vi "Plugin Wrapper Subpanel.vi"() -> ()   [LabVIEW 2021, in "CIF Manager UI.lvlib"]
uses:
  CIF Manager UI.lvlib
  <vilib>/CIF Foundation/CIF Core/CIFUI/Typedef/Run Listen Button.ctl
  CIFManagerUI Class/Typedef/Class Data for Manager SubPanel.ctl
  <vilib>/CIF Foundation/CIF Core/CIFUI/Typedef/Class Data for SubPanel.ctl
  <vilib>/CIF Foundation/CIF Core/CIFUI/Typedef/Core UI References.ctl
  <vilib>/CIF Foundation/CIF Core/CIFUI/Typedef/SubPanel Events.ctl
  <vilib>/CIF Foundation/CIF Core/CIFUI/Typedef/New Connection Plugin Event Data.ctl
  CIFManagerUI Class/Typedef/Core Manager UI References.ctl
  CIFManagerUI Class/Typedef/Channel Connection.ctl
  CIFManagerUI Class/Typedef/New Plugin.ctl
  CIFManagerUI Class/Typedef/CIF_Manager_UI_Tab.ctl
  CIFPluginManager/typedef/New Connection Event Data.ctl
  <vilib>/gRPC/LabVIEW gRPC Library/Shared/grpcId.ctl
  CIFManagerUI Class/CIF_Manager_UI.lvclass/CIF_Manager_UI.ctl
  <vilib>/CIF Foundation/CIF Core/CIFUI/CIF_UI.lvclass/CIF_UI.ctl
  <vilib>/CIF Foundation/CIF Core/CIFUI/Accessors/Read Plugin Connection Map.vi
  <vilib>/CIF Foundation/CIF Core/CIFUI/Accessors/Read Plugin Subpanel Map.vi
  <vilib>/CIF Foundation/CIF Core/CIFUI/SubVIs/Check Run Command Timer.vi
  <vilib>/CIF Foundation/CIF Core/CIFUI/Utilities/Get Human Readable Error.vi
  <vilib>/CIF Foundation/CIF Utilities/Errors/Append Error Location.vi
  <vilib>/CIF Foundation/CIF Core/CIFUI/Accessors/Read Instrument Studio.vi
  CIFManagerUI Class/CIF_Manager_UI.lvclass
  C:/Program Files/National Instruments/LabVIEW 2021/vi.lib/CIF Foundation/CIF Core/CIFUI/CIF_UI.lvclass
  <vilib>/CIF Foundation/CIF Core/CIFUI/UI Helpers/UI Element Update/Empty Tree by Reference.vi
  CIFManagerUI Class/Manager Functions/SubVIs/Initialize Manager Tab by Reference.vi
  <vilib>/CIF Foundation/CIF Core/CIFUI/UI Helpers/UI Element Update/Empty Table by Reference.vi
  CIFManagerUI Class/Wrapper/Close Plugin SubPanel.vi
  <vilib>/CIF Foundation/CIF Utilities/Errors/Human Readable Error Message.vi
  <vilib>/CIF Foundation/CIF Core/CIFUI/CIF_UI.lvclass
  <vilib>/CIF Foundation/CIF Core/CIFCore/Grpc/CIFCoreWrapper/CIFCoreWrapper.lvlib
  <vilib>/gRPC/LabVIEW gRPC Library/grpc-lvsupport-release.lvlib
panel:
  in  "Class Data for Manager SubPanel":T1
  in  "Plugin Selection":u16(ring) items=["tag"]
  in  "Run Listen":T7
  in  "Unload":bool
  in  "Refresh Button":bool
  in  "Plugin Status":string[][](table)
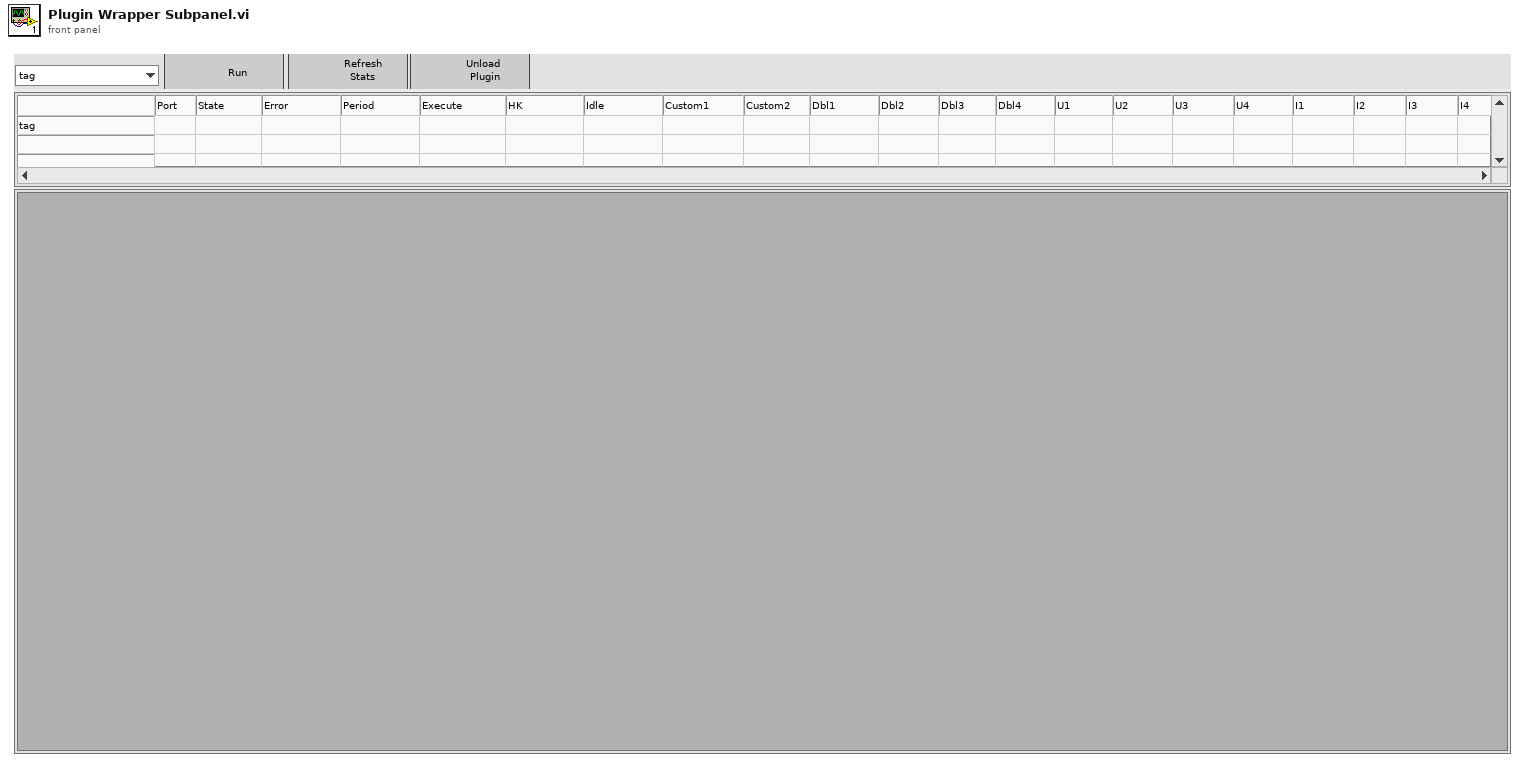
[diagram p1: front panel]
types:
  T1 = typedef "CIF_Manager_UI.lvclass/Class Data for Manager SubPanel.ctl" = cluster{"Class Data for SubPanel":T2, "Manager UI References":T5, "New Manager Connection":refnum<user-event>, "Manager gRPC ID":T6, "Manager Connection":bool}
  T2 = typedef "CIF_UI.lvclass/Class Data for SubPanel.ctl" = cluster{"IP Address":string, "Server Certificate File (.crt)":path, "Connected":bool, "Core UI References":T3, "Subpanel Events":T4, "Manager gRPC Port":u16}
  T3 = typedef "CIF_UI.lvclass/Core UI References.ctl" = cluster{"Plugin Status":refnum<vi>, "Plugin Status Valid":bool, "Connection":refnum<vi>, "Connection Valid":bool, "Exit":refnum<vi>, "Exit Valid":bool, "Run Listen":refnum<vi>, "Run Listen Valid":bool, "Clear Local Error":refnum<vi>, "Clear Local Error Valid":bool, "Local Error":refnum<vi>, "Local Error Valid":bool}
  T4 = typedef "CIF_UI.lvclass/SubPanel Events.ctl" = cluster{"Clear Local Error":refnum<user-event>, "Shutdown":refnum<user-event>, "Plugin Connection":refnum<user-event>}
  T5 = typedef "CIF_Manager_UI.lvclass/Core Manager UI References.ctl" = cluster{"Discovered Plugins":refnum<vi>, "Discovered Plugins Valid":bool, "Loaded Plugins":refnum<vi>, "Loaded Plugins Valid":bool, "Publisher Channels":refnum<vi>, "Publisher Channels Valid":bool, "Subscriber Channels":refnum<vi>, "Subscriber Channels Valid":bool, "Channel Connection":refnum<vi>, "Channel Connection Valid":bool, "New Plugin Load":refnum<vi>, "New Plugin Load Valid":bool, "Errors":refnum<vi>, "Errors Valid":bool, "Plugin to Abort":refnum<vi>, "Plugin to Abort Valid":bool, "CIF Manager Tab":refnum<vi>, "Manger Tab Valid":bool, "System Errors":refnum<vi>, "System Errors Valid":bool, "Plugin Selection":refnum<vi>, "Plugin Selection Valid":bool}
  T6 = typedef "grpc-lvsupport-release.lvlib/grpcId.ctl" = u64
  T7 = typedef "CIF_UI.lvclass/Run Listen Button.ctl" = bool
  T8 = typedef "CIF_UI.lvclass/Plugin Connections.ctl" = cluster{"gRPC ID":T6, "Plugin Info":T9}
  T9 = typedef "CIFCoreCommon.lvlib/PluginInfo.ctl" = cluster{"Name":string, "Type":string, "grpc_port":i32, "Version":T10, "Node Status":T11}
  T10 = typedef "CIFCoreCommon.lvlib/Version Simple.ctl" = cluster{"Major":i32, "Minor":i32, "Fix":i32}
  T11 = typedef "CIFCoreCommon.lvlib/gRPC Reported Plugin Status.ctl" = cluster{"State":T12, "Timing Statistics (us)":T13, "FIFO Statistics (us)":T15, "error":T16, "Monitor Doubles":T17, "Monitor U64":T18, "Monitor I64":T19}
  T12 = typedef "CIFCoreCommon.lvlib/Plugin State.ctl" = enum32{"Null", "Creating", "Listening", "Running", "CleaningUp", "Destroying", "Prepared", "FTE_Run"}
  T13 = typedef "CIFCoreCommon.lvlib/Timing Statistics.ctl" = cluster{"Period":T14, "Wake Error":T14, "Execute":T14, "Housekeep":T14, "Idle":T14, "Cleanup":T14, "Custom 1 (custom units)":T14, "Custom 2 (custom units)":T14}
  T14 = typedef "CIFCoreCommon.lvlib/Timing Stats Base.ctl" = cluster{"Max":i64, "Avg":dbl, "Min":i64}
  T15 = typedef "CIFCoreCommon.lvlib/FIFO Statistics.ctl" = cluster{"From T0":T14, "From Previous Plugin":T14, "Output Error":T14}
  T16 = typedef "CIFCoreCommon.lvlib/Simple Error.ctl" = cluster{"status":bool, "code":i32}
  T17 = typedef "CIFCoreCommon.lvlib/Monitor Doubles.ctl" = cluster{"1":dbl, "2":dbl, "3":dbl, "4":dbl}
  T18 = typedef "CIFCoreCommon.lvlib/Monitor U64.ctl" = cluster{"1":u64, "2":u64, "3":u64, "4":u64}
  T19 = typedef "CIFCoreCommon.lvlib/Monitor I64.ctl" = cluster{"1":i64, "2":i64, "3":i64, "4":i64}
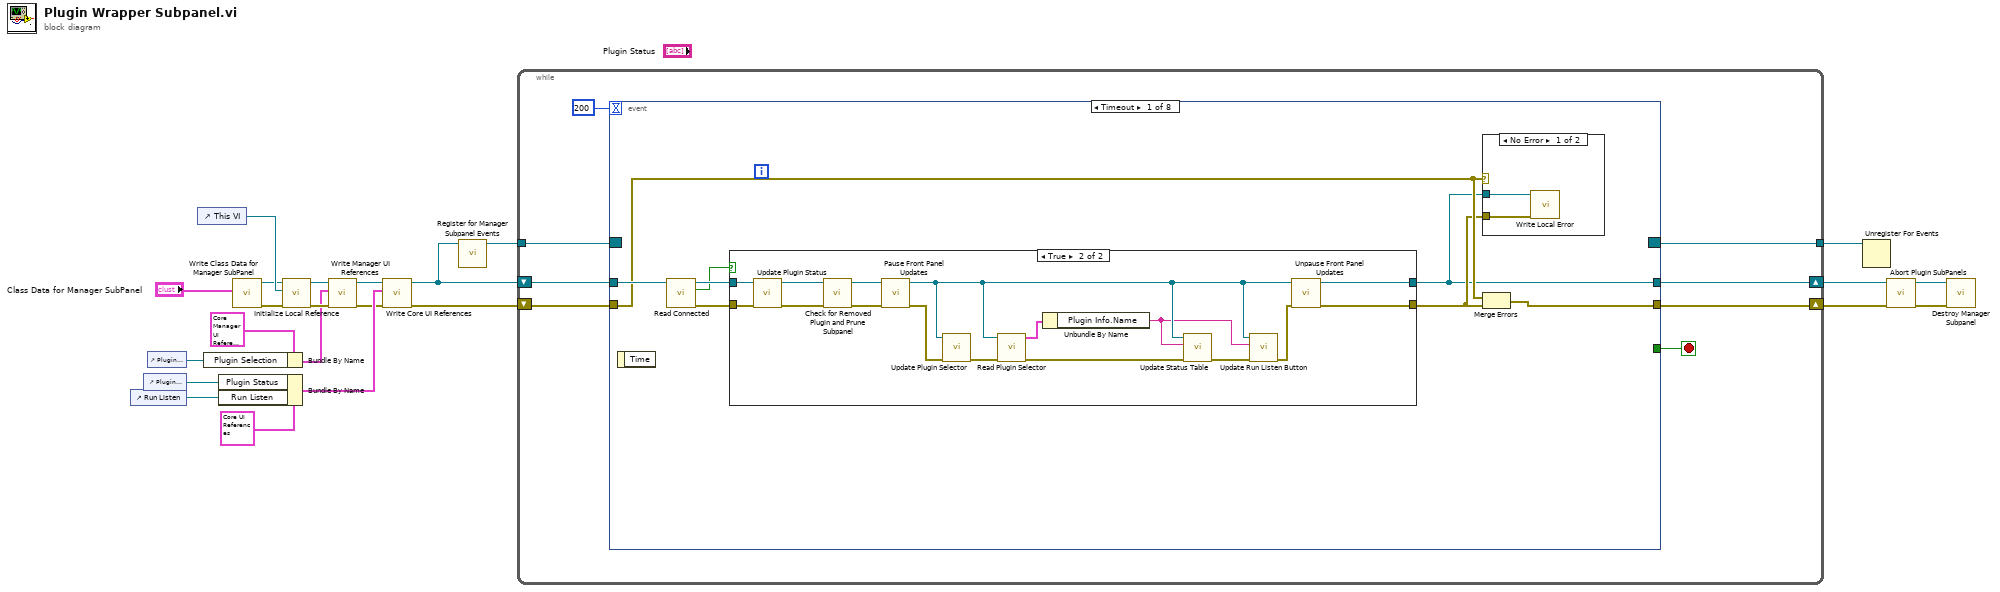
[diagram p0: block diagram]
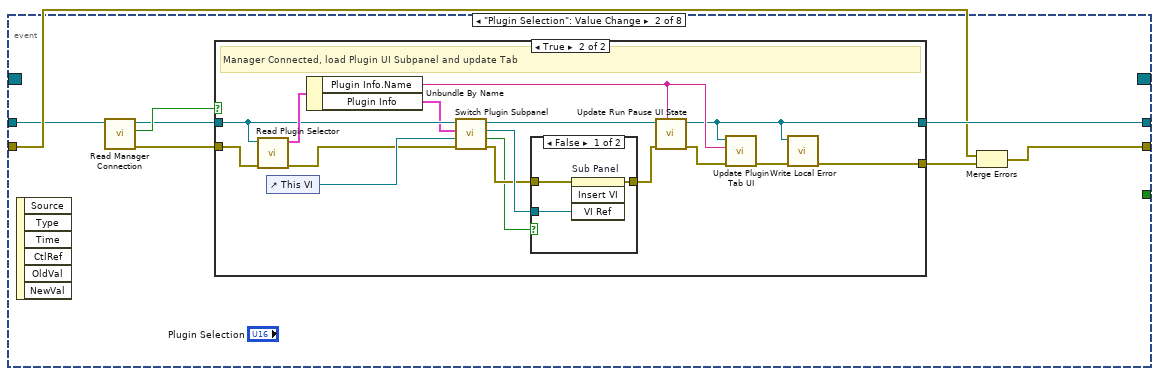
[diagram p4: hidden frame]
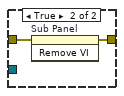
[diagram p6: hidden frame]
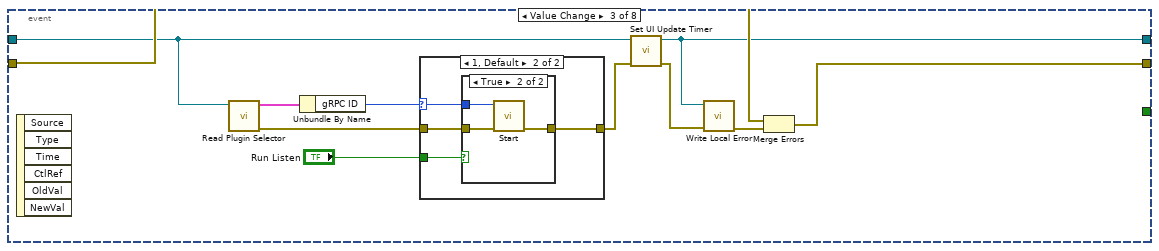
[diagram p7: hidden frame]
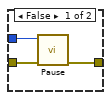
[diagram p9: hidden frame]
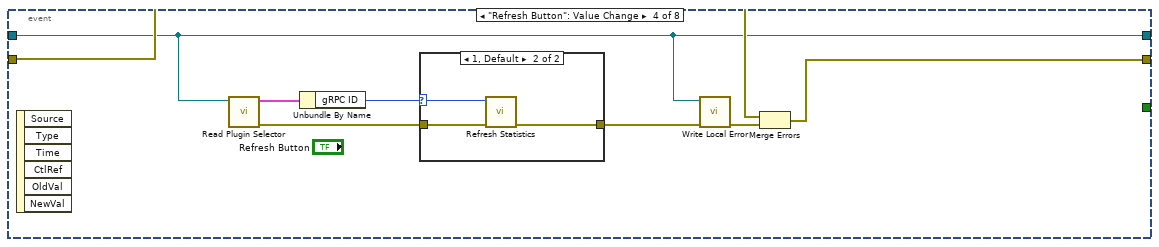
[diagram p10: hidden frame]
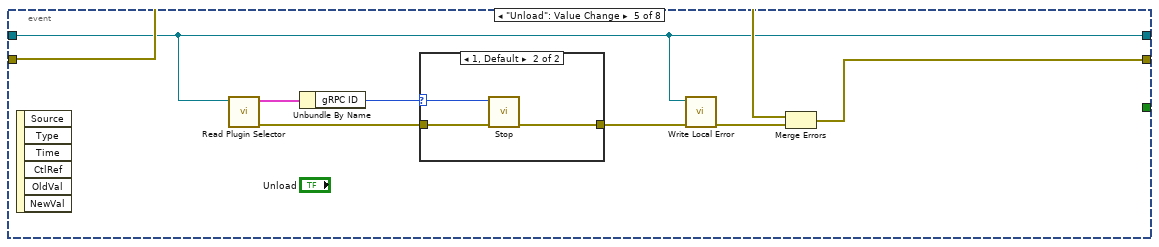
[diagram p12: hidden frame]
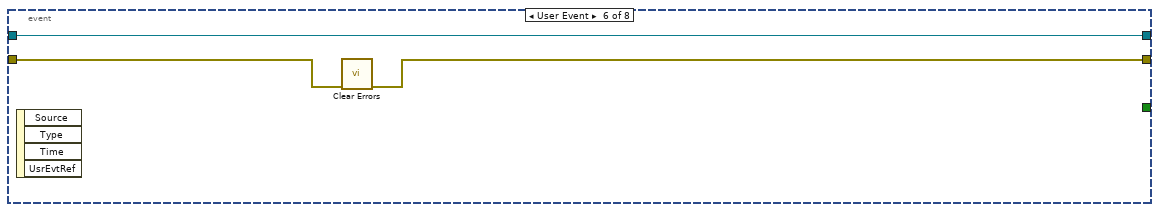
[diagram p14: hidden frame]
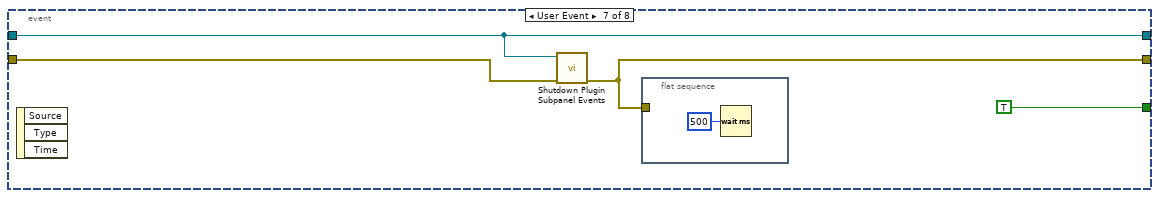
[diagram p15: hidden frame]
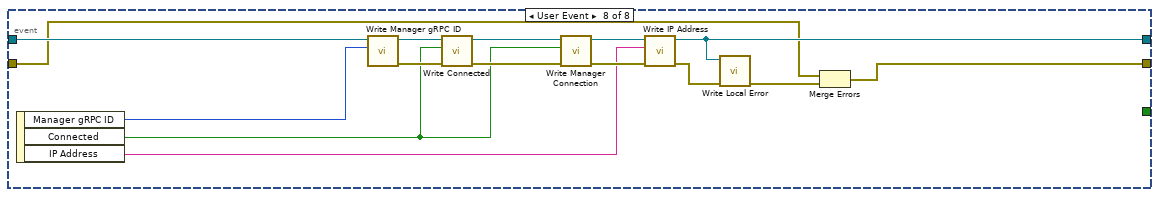
[diagram p16: hidden frame]
diagram:
  n1 = control-ref of="Run Listen"() -> (w19:refnum<vi>)
  n2 = control-ref of="Plugin Status"() -> (w21:refnum<vi>)
  n3 = control-ref of="Plugin Selection"() -> (w17:refnum<vi>)
  n4 = control-ref of="This VI"() -> (w20:refnum<vi>)
  n5 = Bundle By Name(cluster=T5 {"Discovered Plugins"=refnum, "Discovered Plugins Valid"=FALSE, "Loaded Plugins"=refnum, "Loaded Plugins Valid"=FALSE, "Publisher Channels"=refnum, "Publisher Channels Valid"=FALSE, "Subscriber Channels"=refnum, "Subscriber Channels Valid"=FALSE, "Channel Connection"=refnum, "Channel Connection Valid"=FALSE, "New Plugin Load"=refnum, "New Plugin Load Valid"=FALSE, "Errors"=refnum, "Errors Valid"=FALSE, "Plugin to Abort"=refnum, "Plugin to Abort Valid"=FALSE, "CIF Manager Tab"=refnum, "Manger Tab Valid"=FALSE, "System Errors"=refnum, "System Errors Valid"=FALSE, "Plugin Selection"=refnum, "Plugin Selection Valid"=FALSE} ("input cluster"), "Plugin Selection"=w17) -> (w13:T5)
  n6 = Bundle By Name(cluster=T3 {"Plugin Status"=refnum, "Plugin Status Valid"=FALSE, "Connection"=refnum, "Connection Valid"=FALSE, "Exit"=refnum, "Exit Valid"=FALSE, "Run Listen"=refnum, "Run Listen Valid"=FALSE, "Clear Local Error"=refnum, "Clear Local Error Valid"=FALSE, "Local Error"=refnum, "Local Error Valid"=FALSE} ("UI References"), "Plugin Status"=w21, "Run Listen"=w19) -> (w22:T3)
  n7 = call "Write Class Data for Manager SubPanel.vi"("Class Data for Manager SubPanel"="Class Data for Manager SubPanel") -> ("error out"=w5:errorcluster, "CIF_Manager_UI out"=w7:refnum<class "CIF_Manager_UI.lvclass">)  [unwired: 9 in]
  n8 = call <vilib>:"Initialize Local Reference.vi"("error in (no error)"=w5, "This VI"=w20, "CIF_UI in"=w7) -> ("error out"=w15:errorcluster, "CIF_UI out"=w16:refnum<class "CIF_Manager_UI.lvclass">)  [unwired: 7 in]
  n9 = call "Write Manager UI References.vi"("error in (no error)"=w15, "Manager UI References"=w13, "CIF_UI in"=w16) -> ("error out"=w11:errorcluster, "CIF_UI out"=w12:refnum<class "CIF_Manager_UI.lvclass">)  [unwired: 7 in]
  n10 = call <vilib>:"Write Core UI References.vi"("error in (no error)"=w11, "UI References"=w22, "CIF_UI in"=w12) -> ("error out"=w14:errorcluster, "CIF_UI out"=w4:refnum<class "CIF_Manager_UI.lvclass">)  [unwired: 7 in]
  n11 = call "Register for Manager Subpanel Events.vi"("CIF_Manager_UI in"=w4) -> ("Event Registration Refnum"=w3:refnum<event-registration>)  [unwired: 9 in, 1 out]
  n12 = while {
    shift-right: [w27] -> w10
    shift-left: w4 -> [w29]
    shift-right: [w24] -> w9
    shift-left: w14 -> [w28]
    tunnel: w3 -> [w26]
    tunnel: [w25] -> w18
    stop <- w30 stop-if-true
    n13 = event shown="[0] Timeout" {
      selector: w26 -> [_ _ _ _ _ _ _ _]
      dyn-events: [_ _ _ _ _ _ _ _] -> w25
      timeout: 200 -> [_ _ _ _ _ _ _ _]
      tunnel: [_ _ _ _ _ _ TRUE _] -> w30
      tunnel: w29 -> [w36 w61 w94 w113 w125 w137 w142 w153]
      tunnel: w28 -> [w35 w63 w96 w114 w127 w139 w141 w147]
      tunnel: [w33 w62 w95 w115 w126 w138 w140 w146] -> w24
      tunnel: [w32 w64 w93 w113 w125 w137 w142 w148] -> w27
      event Timeout {
        n14 = event-data() -> ()  [unwired: 1 in, 1 out]
        n15 = call <vilib>:"Read Connected.vi"("CIF_UI in"=w36) -> ("error out"=w38:errorcluster, "Connected"=w37:bool, "CIF_UI out"=w39:refnum<class "CIF_Manager_UI.lvclass">)  [unwired: 8 in]
        n16 = case shown="True" w37 {
          tunnel: w38 -> [w42 w59]
          tunnel: [w42 w44] -> w34
          tunnel: w39 -> [w43 w58]
          tunnel: [w43 w45] -> w32
          frame False {
          }
          frame True {
            n17 = call <vilib>:"Update Plugin Status.vi"("error in (no error)"=w59, "CIF_UI in"=w58) -> ("error out"=w55:errorcluster, "CIF_UI out"=w56:refnum<class "CIF_Manager_UI.lvclass">)  [unwired: 8 in]
            n18 = call "Check for Removed Plugin and Prune Subpanel.vi"("error in (no error)"=w55, "CIF_UI in"=w56) -> ("error out"=w53:errorcluster, "CIF_UI out"=w54:refnum<class "CIF_Manager_UI.lvclass">)  [unwired: 8 in]
            n19 = call <vilib>:"Pause Front Panel Updates.vi"("error in (no error)"=w53, "CIF_UI in"=w54) -> ("error out"=w51:errorcluster, "CIF_UI out"=w47:refnum<class "CIF_Manager_UI.lvclass">)  [unwired: 8 in]
            n20 = call "Update Plugin Selector.vi"("error in (no error)"=w51, "CIF_UI in"=w47) -> ("error out"=w52:errorcluster)  [unwired: 9 in]
            n21 = call "Read Plugin Selector.vi"("error in (no error)"=w52, "CIF_UI in"=w47) -> ("error out"=w50:errorcluster, "Plugin Info"=w57:T8)  [unwired: 8 in]
            n22 = Unbundle By Name(w57) -> ("Plugin Info.Name"=w46:string)
            n23 = call <vilib>:"Update Status Table.vi"("error in (no error)"=w50, "Plugin Filter"=w46, "CIFManager_UI in"=w47) -> ("error out"=w49:errorcluster)  [unwired: 8 in]
            n24 = call <vilib>:"Update Run Listen Button.vi"("error in (no error)"=w49, "Plugin Filter"=w46, "CIFManager_UI in"=w47) -> ("error out"=w48:errorcluster)  [unwired: 8 in]
            n25 = call <vilib>:"Unpause Front Panel Updates.vi"("error in (no error)"=w48, "CIF_UI in"=w47) -> ("error out"=w44:errorcluster, "CIF_UI out"=w45:refnum<class "CIF_Manager_UI.lvclass">)  [unwired: 8 in]
          }
        }
        n26 = case shown="No Error" w35 {
          tunnel: w32 -> [w41 _]
          tunnel: w34 -> [w40 _]
          frame No Error {
            n27 = call <vilib>:"Write Local Error.vi"("error in (no error)"=w40, "CIF_UI in"=w41) -> ()  [unwired: 9 in, 1 out]
          }
          frame Error {
          }
        }
        n28 = Merge Errors(w35, w34) -> (w33:errorcluster)
      }
      event "Plugin Selection": Value Change {
        n29 = event-data() -> ()  [unwired: 1 in, 6 out]
        n30 = call <vilib>:"Read Manager Connection.vi"("CIF_UI in"=w61) -> ("error out"=w65:errorcluster, "Manager Connection"=w67:bool, "CIF_UI out"=w66:refnum<class "CIF_Manager_UI.lvclass">)  [unwired: 8 in]
        n31 = case shown="True" w67 {
          tunnel: w65 -> [w68 w85]
          tunnel: w66 -> [w69 w82]
          tunnel: [w69 w74] -> w64
          tunnel: [w68 w73] -> w60
          frame False {
            # "Manager not connected.  Input is not valid. Skip"
          }
          frame True {
            # "Manager Connected, load Plugin UI Subpanel and update Tab"
            n32 = call "Read Plugin Selector.vi"("error in (no error)"=w85, "CIF_UI in"=w82) -> ("error out"=w71:errorcluster, "Plugin Info"=w83:T8)  [unwired: 8 in]
            n33 = control-ref of="This VI"() -> (w76:refnum<vi>)
            n34 = Unbundle By Name(w83) -> ("Plugin Info.Name"=w79:string, "Plugin Info"=w77:T9)
            n35 = call "Switch Plugin Subpanel.vi"("error in (no error)"=w71, "Calling VI"=w76, "Plugin Info"=w77, "CIF_UI in"=w82) -> ("error out"=w72:errorcluster, "Remove Subpanel"=w70:bool, "VI Reference"=w84:refnum<vi>, "CIF_UI out"=w78:refnum<class "CIF_Manager_UI.lvclass">)  [unwired: 4 in]
            n36 = case shown="False" w70 {
              tunnel: w84 -> [w88 _]
              tunnel: [w87 w89] -> w81
              tunnel: w72 -> [w86 w90]
              frame False {
                n37 = invoke on="Sub Panel" class="SubPnl" method="Insert VI"(error in=w86, "VI Ref"=w88) -> (error out=w87:errorcluster)  [unwired: 2 in, 3 out]
              }
              frame True {
                n38 = invoke on="Sub Panel" class="SubPnl" method="Remove VI"(error in=w90) -> (error out=w89:errorcluster)  [unwired: 2 in, 2 out]
              }
            }
            n39 = call <vilib>:"Update Run Pause UI State.vi"("Plugin Name"=w79, "error in (no error)"=w81, "CIF_UI in"=w78) -> ("error out"=w80:errorcluster, "CIF_UI out"=w74:refnum<class "CIF_Manager_UI.lvclass">)  [unwired: 7 in]
            n40 = call "Update Plugin Tab UI.vi"("error in (no error)"=w80, "Plugin Name"=w79, "CIF_UI in"=w74) -> ("error out"=w75:errorcluster)  [unwired: 8 in]
            n41 = call <vilib>:"Write Local Error.vi"("error in (no error)"=w75, "CIF_UI in"=w74) -> ("error out"=w73:errorcluster)  [unwired: 9 in]
          }
        }
        n42 = Merge Errors(w63, w60) -> (w62:errorcluster)
      }
      event Value Change {
        n43 = event-data() -> ()  [unwired: 1 in, 6 out]
        n44 = call "Read Plugin Selector.vi"("CIF_UI in"=w94) -> ("error out"=w99:errorcluster, "Plugin Info"=w101:T8)  [unwired: 9 in]
        n45 = Unbundle By Name(w101) -> ("gRPC ID"=w100:T6)
        n46 = case shown="1, Default" w100 {
          selector: w100 -> [_ w106]
          tunnel: w99 -> [w102 w105]
          tunnel: "Run Listen" -> [_ w104]
          tunnel: [w102 w103] -> w92
          frame 0 {
          }
          frame 1, Default {
            n47 = case shown="True" w104 {
              tunnel: w106 -> [w109 w112]
              tunnel: w105 -> [w108 w111]
              tunnel: [w107 w110] -> w103
              frame False {
                n48 = call <vilib>:"Pause.vi"("error in"=w108, "gRPC ID"=w109) -> ("error out"=w107:errorcluster)  [unwired: 8 in, 1 out]
              }
              frame True {
                n49 = call <vilib>:"Start.vi"("error in"=w111, "gRPC ID"=w112) -> ("error out"=w110:errorcluster)  [unwired: 8 in, 1 out]
              }
            }
          }
        }
        n50 = call "Set UI Update Timer.vi"("error in (no error)"=w92, "CIF_UI in"=w94) -> ("error out"=w91:errorcluster, "CIF_UI out"=w93:refnum<class "CIF_Manager_UI.lvclass">)  [unwired: 8 in]
        n51 = call <vilib>:"Write Local Error.vi"("error in (no error)"=w91, "CIF_UI in"=w93) -> ("error out"=w97:errorcluster)  [unwired: 9 in]
        n52 = Merge Errors(w96, w97) -> (w95:errorcluster)
      }
      event "Refresh Button": Value Change {
        n53 = event-data() -> ()  [unwired: 1 in, 6 out]
        n54 = call "Read Plugin Selector.vi"("CIF_UI in"=w113) -> ("error out"=w118:errorcluster, "Plugin Info"=w120:T8)  [unwired: 9 in]
        n55 = Unbundle By Name(w120) -> ("gRPC ID"=w119:T6)
        n56 = case shown="1, Default" w119 {
          selector: w119 -> [_ w124]
          tunnel: w118 -> [w121 w123]
          tunnel: [w121 w122] -> w117
          frame 0 {
          }
          frame 1, Default {
            n57 = call <vilib>:"Refresh Statistics.vi"("error in"=w123, "gRPC ID"=w124) -> ("error out"=w122:errorcluster)  [unwired: 8 in, 1 out]
          }
        }
        n58 = call <vilib>:"Write Local Error.vi"("error in (no error)"=w117, "CIF_UI in"=w113) -> ("error out"=w116:errorcluster)  [unwired: 9 in]
        n59 = Merge Errors(w114, w116) -> (w115:errorcluster)
      }
      event "Unload": Value Change {
        n60 = event-data() -> ()  [unwired: 1 in, 6 out]
        n61 = call "Read Plugin Selector.vi"("CIF_UI in"=w125) -> ("error out"=w130:errorcluster, "Plugin Info"=w132:T8)  [unwired: 9 in]
        n62 = Unbundle By Name(w132) -> ("gRPC ID"=w131:T6)
        n63 = case shown="1, Default" w131 {
          selector: w131 -> [_ w134]
          tunnel: w130 -> [w133 w136]
          tunnel: [w133 w135] -> w129
          frame 0 {
          }
          frame 1, Default {
            n64 = call <vilib>:"Stop.vi"("error in"=w136, "gRPC ID"=w134) -> ("error out"=w135:errorcluster)  [unwired: 8 in, 1 out]
          }
        }
        n65 = call <vilib>:"Write Local Error.vi"("error in (no error)"=w129, "CIF_UI in"=w125) -> ("error out"=w128:errorcluster)  [unwired: 9 in]
        n66 = Merge Errors(w127, w128) -> (w126:errorcluster)
      }
      event User Event {
        n67 = event-data() -> ()  [unwired: 1 in, 4 out]
        n68 = call <vilib>:"Clear Errors.vi"("error in (no error)"=w139) -> ("error out"=w138:errorcluster)  [unwired: 5 in, 1 out]
      }
      event User Event {
        n69 = event-data() -> ()  [unwired: 1 in, 3 out]
        n70 = call <vilib>:"Shutdown Plugin Subpanel Events.vi"("error in (no error)"=w141, "CIF_UI in"=w142) -> ("error out"=w140:errorcluster)  [unwired: 9 in]
        n71 = flat-sequence {
          tunnel: w140 -> [_]
          frame #0 {
            n72 = Wait (ms)(milliseconds to wait=u32 500) -> ()  [unwired: 1 out]
          }
        }
      }
      event User Event {
        n73 = event-data() -> ("Manager gRPC ID"=w150:T6, "Connected"=w151:bool, "IP Address"=w152:string)  [unwired: 1 in]
        n74 = call <vilib>:"Write Manager gRPC ID.vi"("gRPCid"=w150, "CIF_UI in"=w153) -> ("error out"=w158:errorcluster, "CIF_UI out"=w159:refnum<class "CIF_Manager_UI.lvclass">)  [unwired: 8 in]
        n75 = call <vilib>:"Write Connected.vi"("error in (no error)"=w158, "Connected"=w151, "CIF_UI in"=w159) -> ("error out"=w156:errorcluster, "CIF_UI out"=w157:refnum<class "CIF_Manager_UI.lvclass">)  [unwired: 7 in]
        n76 = call <vilib>:"Write Manager Connection.vi"("error in (no error)"=w156, "Manager Connection"=w151, "CIF_UI in"=w157) -> ("error out"=w154:errorcluster, "CIF_UI out"=w155:refnum<class "CIF_Manager_UI.lvclass">)  [unwired: 7 in]
        n77 = call <vilib>:"Write IP Address.vi"("error in (no error)"=w154, "IP Address"=w152, "CIF_UI in"=w155) -> ("error out"=w149:errorcluster, "CIF_UI out"=w148:refnum<class "CIF_Manager_UI.lvclass">)  [unwired: 7 in]
        n78 = call <vilib>:"Write Local Error.vi"("error in (no error)"=w149, "CIF_UI in"=w148) -> ("error out"=w145:errorcluster)  [unwired: 9 in]
        n79 = Merge Errors(w147, w145) -> (w146:errorcluster)
      }
    }
  }
  n80 = Unregister For Events(event registration refnum=w18) -> ()  [unwired: 1 in, 1 out]
  n81 = call <vilib>:"Abort Plugin SubPanels.vi"("error in (no error)"=w9, "CIF_UI in"=w10) -> ("error out"=w1:errorcluster, "CIF_UI out"=w2:refnum<class "CIF_Manager_UI.lvclass">)  [unwired: 8 in]
  n82 = call "Destroy Manager Subpanel.vi"("error in (no error)"=w1, "CIF_Manager_UI in"=w2) -> ()  [unwired: 8 in, 2 out]
